vi "Swerve Begin.vi"() -> ()   [LabVIEW 2016]
uses:
  <vilib>/Rock Robotics/WPI/ThirdParty/CanMotor/TalonSRX/WPI_CANTalonSRX_APIControlMode.ctl
  <vilib>/Rock Robotics/WPI/ThirdParty/CanMotor/TalonSRX/WPI_CANTalonSRX_APIFeedbackSelect.ctl
  <vilib>/Rock Robotics/SystemInterfaces/DIO/FPGA_DIOPWMChannel.ctl
  <vilib>/Rock Robotics/WPI/MotorControl/WPI_MotorControlOpen VictorSP.vi
panel:
  in  "Reverse Peak Output":dbl=-1.0
  in  "Forward Peak Output":dbl=1.0
  in  "Allowable Closed-Loop Error":u16
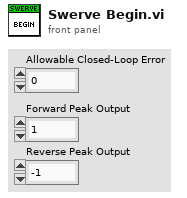
[diagram p1: front panel]
types:
  T1 = typedef "WPI_CANTalonSRX_APIFeedbackSelect.ctl" = enum16{"Digital Quadrature Encoder", "Analog Potentiometer", "Analog Encoder", "Count on Quad-A (Rising-Edge)", "Count on Quad-A (Falling-Edge)", "CTR Magnetic Enc (Absolute)", "CTR Magnetic Enc (Relative)", "Pulse Width"}
  T2 = typedef "WPI_CANTalonSRX_APIControlMode.ctl" = enum8{"Percent VBus", "Speed", "Position", "Slave", "Unchanged / Invalid", "Voltage Compensation", "Current", "Motion Profile", "Motion Magic"}
  T3 = typedef "FPGA_DIOPWMChannel.ctl" = enum8{"PWM 0", "PWM 1", "PWM 2", "PWM 3", "PWM 4", "PWM 5", "PWM 6", "PWM 7", "PWM 8", "PWM 9", "PWM MXP 0", "PWM MXP 1", "PWM MXP 2", "PWM MXP 3", "PWM MXP 4", "PWM MXP 5", "PWM MXP 6", "PWM MXP 7", "PWM MXP 8", "PWM MXP 9", "Invalid"}
  T4 = typedef "WPI_MotorControlDeviceRef.ctl" = cluster{"DeviceStatus":errorcluster, "Type":T5, "PWM":cluster{"PWM Channel":T3, "DeadBand":T6}, "CAN":cluster{"Device Number":u8, "SetOutput VI Ref":variant, "GetOutput VI Ref":variant, "Enable VI Ref":variant, "Disable VI Ref":variant, "Data":variant}, "Invert":bool}
  T5 = typedef "WPI_MotorControlType.ctl" = enum16{"PWM", "CAN"}
  T6 = typedef "WPI_PWMDeadband.ctl" = cluster{"Name":string, "maxPositivePwm":i32, "minPositivePwm":i32, "centerPwm":i32, "maxNegativePwm":i32, "minNegativePwm":i32, "angularRange":u16}
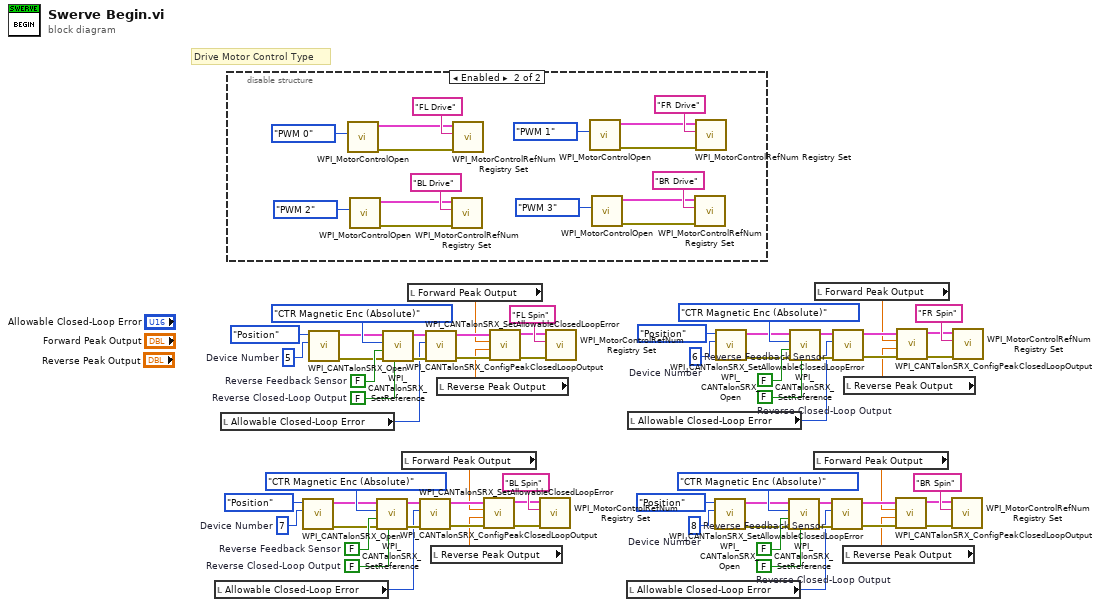
[diagram p0: block diagram]
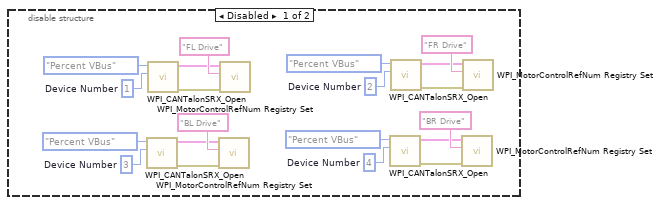
[diagram p2: hidden frame]
diagram:
  w12 = FALSE  # Reverse Closed-Loop Output
  w13 = FALSE  # Reverse Feedback Sensor
  w15 = u8 8  # Device Number
  w29 = FALSE  # Reverse Closed-Loop Output
  w30 = FALSE  # Reverse Feedback Sensor
  w32 = u8 7  # Device Number
  w46 = FALSE  # Reverse Closed-Loop Output
  w47 = FALSE  # Reverse Feedback Sensor
  w49 = u8 6  # Device Number
  w63 = FALSE  # Reverse Closed-Loop Output
  w64 = FALSE  # Reverse Feedback Sensor
  w66 = u8 5  # Device Number
  # "Drive Motor Control Type"
  n1 = local read "Allowable Closed-Loop Error"() -> (w20:u16)
  n2 = local read "Allowable Closed-Loop Error"() -> (w54:u16)
  n3 = disable-structure shown="Enabled" {
    frame Disabled {
      w71 = u8 4  # Device Number
      w76 = u8 3  # Device Number
      w81 = u8 2  # Device Number
      w86 = u8 1  # Device Number
      n4 = call <vilib>:"WPI_CANTalonSRX_Open.vi"("Device Number"=w76, "Control Mode"=WPI_CANTalonSRX_APIControlMode."Percent VBus") -> ("error out"=w74:errorcluster, "CAN Talon SRX Ref"=w75:T4)  [unwired: 8 in]
      n5 = call <vilib>:"WPI_CANTalonSRX_Open.vi"("Device Number"=w86, "Control Mode"=WPI_CANTalonSRX_APIControlMode."Percent VBus") -> ("error out"=w84:errorcluster, "CAN Talon SRX Ref"=w85:T4)  [unwired: 8 in]
      n6 = call <vilib>:"WPI_MotorControlRefNum Registry Set.vi"("error in (no error)"=w74, "refnum name"="BL Drive", "MotorControlDevRef"=w75) -> ()  [unwired: 7 in, 2 out]
      n7 = call <vilib>:"WPI_MotorControlRefNum Registry Set.vi"("error in (no error)"=w84, "refnum name"="FL Drive", "MotorControlDevRef"=w85) -> ()  [unwired: 7 in, 2 out]
      n8 = call <vilib>:"WPI_CANTalonSRX_Open.vi"("Device Number"=w71, "Control Mode"=WPI_CANTalonSRX_APIControlMode."Percent VBus") -> ("error out"=w69:errorcluster, "CAN Talon SRX Ref"=w70:T4)  [unwired: 8 in]
      n9 = call <vilib>:"WPI_CANTalonSRX_Open.vi"("Device Number"=w81, "Control Mode"=WPI_CANTalonSRX_APIControlMode."Percent VBus") -> ("error out"=w79:errorcluster, "CAN Talon SRX Ref"=w80:T4)  [unwired: 8 in]
      n10 = call <vilib>:"WPI_MotorControlRefNum Registry Set.vi"("error in (no error)"=w69, "refnum name"="BR Drive", "MotorControlDevRef"=w70) -> ()  [unwired: 7 in, 2 out]
      n11 = call <vilib>:"WPI_MotorControlRefNum Registry Set.vi"("error in (no error)"=w79, "refnum name"="FR Drive", "MotorControlDevRef"=w80) -> ()  [unwired: 7 in, 2 out]
    }
    frame Enabled {
      n12 = call-poly <vilib>:"WPI_MotorControlOpen.vi"("PWM Channel"=FPGA_DIOPWMChannel."PWM 0") -> ("error out"=w99:errorcluster, "MotorControlDeviceRef"=w100:T4)  [unwired: 9 in]
      n13 = call-poly <vilib>:"WPI_MotorControlOpen.vi"("PWM Channel"=FPGA_DIOPWMChannel."PWM 2") -> ("error out"=w93:errorcluster, "MotorControlDeviceRef"=w94:T4)  [unwired: 9 in]
      n14 = call <vilib>:"WPI_MotorControlRefNum Registry Set.vi"("error in (no error)"=w93, "refnum name"="BL Drive", "MotorControlDevRef"=w94) -> ()  [unwired: 7 in, 2 out]
      n15 = call <vilib>:"WPI_MotorControlRefNum Registry Set.vi"("error in (no error)"=w99, "refnum name"="FL Drive", "MotorControlDevRef"=w100) -> ()  [unwired: 7 in, 2 out]
      n16 = call-poly <vilib>:"WPI_MotorControlOpen.vi"("PWM Channel"=FPGA_DIOPWMChannel."PWM 1") -> ("error out"=w89:errorcluster, "MotorControlDeviceRef"=w90:T4)  [unwired: 9 in]
      n17 = call-poly <vilib>:"WPI_MotorControlOpen.vi"("PWM Channel"=FPGA_DIOPWMChannel."PWM 3") -> ("error out"=w91:errorcluster, "MotorControlDeviceRef"=w92:T4)  [unwired: 9 in]
      n18 = call <vilib>:"WPI_MotorControlRefNum Registry Set.vi"("error in (no error)"=w91, "refnum name"="BR Drive", "MotorControlDevRef"=w92) -> ()  [unwired: 7 in, 2 out]
      n19 = call <vilib>:"WPI_MotorControlRefNum Registry Set.vi"("error in (no error)"=w89, "refnum name"="FR Drive", "MotorControlDevRef"=w90) -> ()  [unwired: 7 in, 2 out]
    }
  }
  n20 = call <vilib>:"WPI_CANTalonSRX_Open.vi"("Device Number"=w32, "Control Mode"=WPI_CANTalonSRX_APIControlMode."Position") -> ("error out"=w27:errorcluster, "CAN Talon SRX Ref"=w28:T4)  [unwired: 8 in]
  n21 = call <vilib>:"WPI_CANTalonSRX_Open.vi"("Device Number"=w66, "Control Mode"=WPI_CANTalonSRX_APIControlMode."Position") -> ("error out"=w61:errorcluster, "CAN Talon SRX Ref"=w62:T4)  [unwired: 8 in]
  n22 = call <vilib>:"WPI_CANTalonSRX_SetReference.vi"("Reverse Closed-Loop Output"=w29, "error in (no error)"=w27, "Reverse Feedback Sensor"=w30, "Feedback Reference"=WPI_CANTalonSRX_APIFeedbackSelect."CTR Magnetic Enc (Absolute)", "CAN Talon SRX Ref"=w28) -> ("error out"=w25:errorcluster, "CAN Talon SRX Ref"=w26:T4)  [unwired: 5 in]
  n23 = call <vilib>:"WPI_CANTalonSRX_SetReference.vi"("Reverse Closed-Loop Output"=w63, "error in (no error)"=w61, "Reverse Feedback Sensor"=w64, "Feedback Reference"=WPI_CANTalonSRX_APIFeedbackSelect."CTR Magnetic Enc (Absolute)", "CAN Talon SRX Ref"=w62) -> ("error out"=w59:errorcluster, "CAN Talon SRX Ref"=w60:T4)  [unwired: 5 in]
  n24 = local read "Forward Peak Output"() -> (w19:dbl)
  n25 = local read "Forward Peak Output"() -> (w53:dbl)
  n26 = call <vilib>:"WPI_CANTalonSRX_SetAllowableClosedLoopError.vi"("error in (no error)"=w25, "Allowable Closed-Loop Error"=w20, "CAN Talon SRX Ref"=w26) -> ("error out"=w24:errorcluster, "CAN Talon SRX Ref"=w23:T4)  [unwired: 7 in]
  n27 = call <vilib>:"WPI_CANTalonSRX_SetAllowableClosedLoopError.vi"("error in (no error)"=w59, "Allowable Closed-Loop Error"=w54, "CAN Talon SRX Ref"=w60) -> ("error out"=w58:errorcluster, "CAN Talon SRX Ref"=w57:T4)  [unwired: 7 in]
  n28 = local read "Reverse Peak Output"() -> (w18:dbl)
  n29 = local read "Reverse Peak Output"() -> (w52:dbl)
  n30 = call <vilib>:"WPI_CANTalonSRX_ConfigPeakClosedLoopOutput.vi"("error in (no error)"=w24, "Reverse Peak Output"=w18, "Forward Peak Output"=w19, "CAN Talon SRX Ref"=w23) -> ("error out"=w21:errorcluster, "CAN Talon SRX Ref"=w22:T4)  [unwired: 6 in]
  n31 = call <vilib>:"WPI_CANTalonSRX_ConfigPeakClosedLoopOutput.vi"("error in (no error)"=w58, "Reverse Peak Output"=w52, "Forward Peak Output"=w53, "CAN Talon SRX Ref"=w57) -> ("error out"=w55:errorcluster, "CAN Talon SRX Ref"=w56:T4)  [unwired: 6 in]
  n32 = call <vilib>:"WPI_MotorControlRefNum Registry Set.vi"("error in (no error)"=w21, "refnum name"="BL Spin", "MotorControlDevRef"=w22) -> ()  [unwired: 7 in, 2 out]
  n33 = call <vilib>:"WPI_MotorControlRefNum Registry Set.vi"("error in (no error)"=w55, "refnum name"="FL Spin", "MotorControlDevRef"=w56) -> ()  [unwired: 7 in, 2 out]
  n34 = local read "Allowable Closed-Loop Error"() -> (w3:u16)
  n35 = local read "Allowable Closed-Loop Error"() -> (w37:u16)
  n36 = call <vilib>:"WPI_CANTalonSRX_Open.vi"("Device Number"=w15, "Control Mode"=WPI_CANTalonSRX_APIControlMode."Position") -> ("error out"=w10:errorcluster, "CAN Talon SRX Ref"=w11:T4)  [unwired: 8 in]
  n37 = call <vilib>:"WPI_CANTalonSRX_Open.vi"("Device Number"=w49, "Control Mode"=WPI_CANTalonSRX_APIControlMode."Position") -> ("error out"=w44:errorcluster, "CAN Talon SRX Ref"=w45:T4)  [unwired: 8 in]
  n38 = call <vilib>:"WPI_CANTalonSRX_SetReference.vi"("Reverse Closed-Loop Output"=w12, "error in (no error)"=w10, "Reverse Feedback Sensor"=w13, "Feedback Reference"=WPI_CANTalonSRX_APIFeedbackSelect."CTR Magnetic Enc (Absolute)", "CAN Talon SRX Ref"=w11) -> ("error out"=w8:errorcluster, "CAN Talon SRX Ref"=w9:T4)  [unwired: 5 in]
  n39 = call <vilib>:"WPI_CANTalonSRX_SetReference.vi"("Reverse Closed-Loop Output"=w46, "error in (no error)"=w44, "Reverse Feedback Sensor"=w47, "Feedback Reference"=WPI_CANTalonSRX_APIFeedbackSelect."CTR Magnetic Enc (Absolute)", "CAN Talon SRX Ref"=w45) -> ("error out"=w42:errorcluster, "CAN Talon SRX Ref"=w43:T4)  [unwired: 5 in]
  n40 = local read "Forward Peak Output"() -> (w2:dbl)
  n41 = local read "Forward Peak Output"() -> (w36:dbl)
  n42 = call <vilib>:"WPI_CANTalonSRX_SetAllowableClosedLoopError.vi"("error in (no error)"=w8, "Allowable Closed-Loop Error"=w3, "CAN Talon SRX Ref"=w9) -> ("error out"=w7:errorcluster, "CAN Talon SRX Ref"=w6:T4)  [unwired: 7 in]
  n43 = call <vilib>:"WPI_CANTalonSRX_SetAllowableClosedLoopError.vi"("error in (no error)"=w42, "Allowable Closed-Loop Error"=w37, "CAN Talon SRX Ref"=w43) -> ("error out"=w41:errorcluster, "CAN Talon SRX Ref"=w40:T4)  [unwired: 7 in]
  n44 = local read "Reverse Peak Output"() -> (w1:dbl)
  n45 = local read "Reverse Peak Output"() -> (w35:dbl)
  n46 = call <vilib>:"WPI_CANTalonSRX_ConfigPeakClosedLoopOutput.vi"("error in (no error)"=w7, "Reverse Peak Output"=w1, "Forward Peak Output"=w2, "CAN Talon SRX Ref"=w6) -> ("error out"=w4:errorcluster, "CAN Talon SRX Ref"=w5:T4)  [unwired: 6 in]
  n47 = call <vilib>:"WPI_CANTalonSRX_ConfigPeakClosedLoopOutput.vi"("error in (no error)"=w41, "Reverse Peak Output"=w35, "Forward Peak Output"=w36, "CAN Talon SRX Ref"=w40) -> ("error out"=w38:errorcluster, "CAN Talon SRX Ref"=w39:T4)  [unwired: 6 in]
  n48 = call <vilib>:"WPI_MotorControlRefNum Registry Set.vi"("error in (no error)"=w4, "refnum name"="BR Spin", "MotorControlDevRef"=w5) -> ()  [unwired: 7 in, 2 out]
  n49 = call <vilib>:"WPI_MotorControlRefNum Registry Set.vi"("error in (no error)"=w38, "refnum name"="FR Spin", "MotorControlDevRef"=w39) -> ()  [unwired: 7 in, 2 out]
